vi "LVLibNameFromFileName.vi"(11 "VI Name / CTL Name / LVCLASS Name":string) -> (3 "Library Name":string)   [LabVIEW 2019, in "DepsWatch.lvlib"]
uses:
  DepsWatch.lvlib
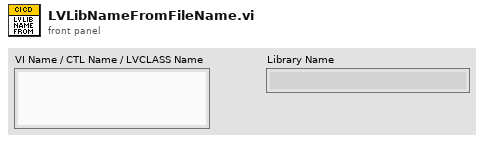
[diagram p1: front panel]
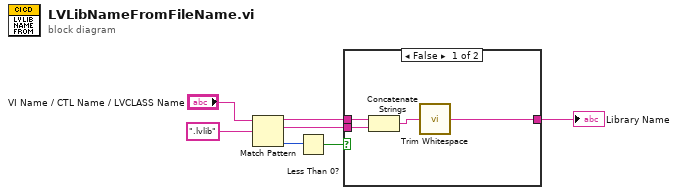
[diagram p0: block diagram]
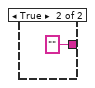
[diagram p2: hidden frame]
diagram:
  n1 = Match Pattern(string="VI Name / CTL Name / LVCLASS Name", regular expression=".lvlib") -> (before substring=w5:string, match substring=w4:string, offset past match=w2:i32)  [unwired: 1 in, 1 out]
  n2 = Less Than 0?(x=w2) -> (x < 0?=w1:bool)
  n3 = case shown="False" w1 {
    tunnel: w5 -> [w11 _]
    tunnel: w4 -> [w10 _]
    tunnel: [w8 "" ("trimmed string")] -> w3
    frame False {
      n4 = Concatenate Strings(w11, w10) -> (w9:string)
      n5 = call <vilib>:"Trim Whitespace.vi"("string"=w9) -> ("trimmed string"=w8:string)  [unwired: 1 in]
    }
    frame True {
    }
  }
  "Library Name" <- w3
